vi "Set Detailed Help URL.vi"(6 "Path Tokens":string[](array[string]), 8 "Error In":errorcluster, 9 "Page Name":string, 10 "Wik Help Base URL":string="https://www.labviewmakerhub.com/doku.php?id=learn:libraries:linx:reference:labview:", 11 "VI Refnum":refnum<vi>) -> (0 "Error Out":errorcluster, 3 "VI Refnum":refnum<vi>)   [LabVIEW 2014]
doc: "test"
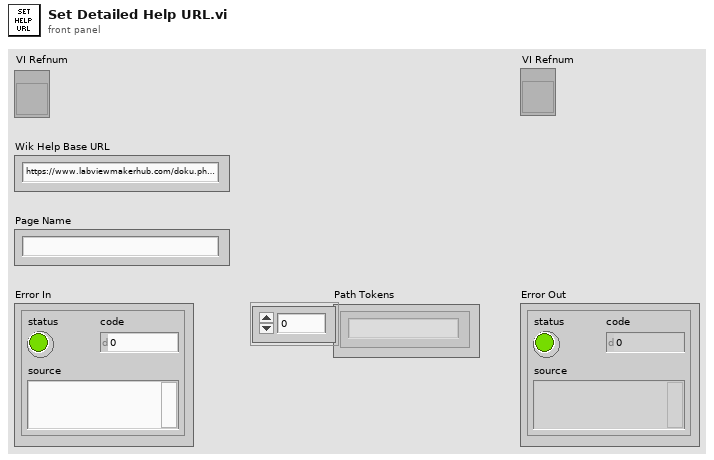
[diagram p1: front panel]
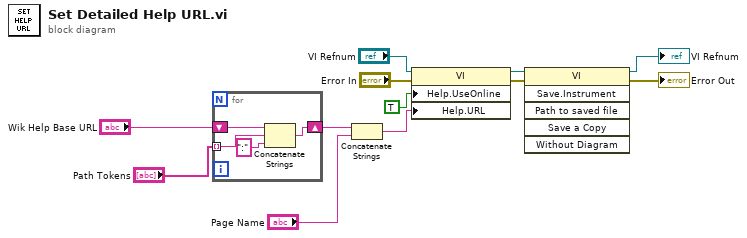
[diagram p0: block diagram]
diagram:
  n1 = for {
    shift-right: [w13] -> w7
    shift-left: "Wik Help Base URL" -> [w16]
    tunnel: "Path Tokens" -> [w15] mode=indexing
    n2 = Concatenate Strings(w16, w15, ":" ("string")) -> (w13:string)
  }
  n3 = Concatenate Strings(w7, "Page Name") -> (w5:string)
  n4 = property class="VI"(reference="VI Refnum", error in="Error In", "Help.UseOnline"=TRUE ("Help:Use Web URL"), "Help.URL"=w5) -> (reference out=w3:refnum<vi>, error out=w4:errorcluster)
  n5 = invoke class="VI" method="Save.Instrument"(reference=w3, error in=w4) -> (reference out=→"VI Refnum":refnum<vi>, error out=→"Error Out":errorcluster)  [unwired: 4 in, 4 out]
